vi "Pose3d_getXYZ.vi"(11 "in Pose3d":T1={"Translation3d"={"X"=0.0, "Y"=0.0, "Z"=0.0}, "Rotation3d"={"Q_quaternion"={"R"=1.0, "V"=[0.0, 0.0, 0.0]}}} {"Translation3d"."Z" format="%14.3f"; "Translation3d"."Y" format="%14.3f"; "Translation3d"."X" format="%14.3f"}) -> (1 "Z":dbl, 2 "Y":dbl, 3 "X":dbl)   [LabVIEW 2019, in "Trajectory_Library.lvlib"]
doc: "Returns the X, Y, Z elements of the translation component of the transformation.\n\nParmeters:\n- IN POSE3D - The POSE data structure\n\nRETURNS:\n - X - The X element of the translational component of the pose.\n - Y - The Y element of the translational component of the pose.\n - Z - The Z element of the translational component of the pose."
uses:
  Trajectory_Library.lvlib
  TypeDef/TRANSLATION3D.ctl
  TypeDef/QUATERNION.ctl
  TypeDef/ROTATION3D.ctl
  TypeDef/POSE3D.ctl
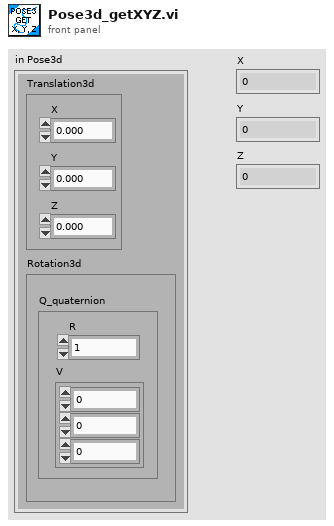
[diagram p1: front panel]
types:
  T1 = typedef "Trajectory_Library.lvlib/POSE3D.ctl" = cluster{"Translation3d":T2, "Rotation3d":T3}
  T2 = typedef "Trajectory_Library.lvlib/TRANSLATION3D.ctl" = cluster{"X":dbl, "Y":dbl, "Z":dbl}
  T3 = typedef "Trajectory_Library.lvlib/ROTATION3D.ctl" = cluster{"Q_quaternion":T4}
  T4 = typedef "Trajectory_Library.lvlib/QUATERNION.ctl" = cluster{"R":dbl, "V":dbl[]}
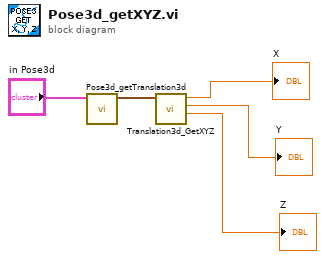
[diagram p0: block diagram]
diagram:
  n1 = call "Pose3d_getTranslation3d.vi"("in Pose3d"="in Pose3d") -> ("out Translation3d"=w4:T2)  [unwired: 10 in]
  n2 = call "Translation3d_GetXYZ.vi"("In Translation3d"=w4) -> ("Z"=→"Z":dbl, "Y"=→"Y":dbl, "X"=→"X":dbl)  [unwired: 8 in]
